vi "animate side opening.vi"(10 "expand/collapse":bool, 11 "Splitter in":refnum<vi>) -> ()   [LabVIEW 2016, in "FPGA RM System Definition API.lvlib"]
uses:
  FPGA-Resource-Manager-APIs/Source/System Definition/FPGA RM System Definition API.lvlib
  visualizer globals.vi
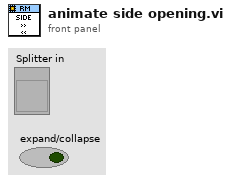
[diagram p1: front panel]
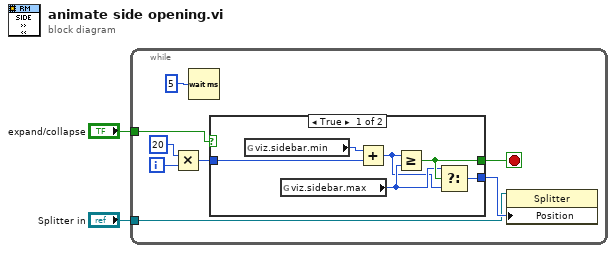
[diagram p0: block diagram]
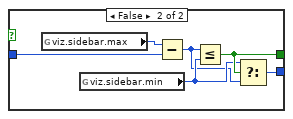
[diagram p2: hidden frame]
diagram:
  n1 = while {
    tunnel: "expand/collapse" -> [w10]
    tunnel: "Splitter in" -> [w3]
    i -> [w6]
    stop <- w9 stop-if-true
    n2 = Multiply(x=20, y=w6) -> (x*y=w5:i32)
    n3 = Wait (ms)(milliseconds to wait=u32 5) -> ()  [unwired: 1 out]
    n4 = case shown="True" w10 {
      tunnel: [w14 w20] -> w9
      tunnel: [w11 w17] -> w8
      tunnel: w5 -> [w16 w22]
      frame True {
        n5 = global read "visualizer globals.vi" "viz.sidebar.min"() -> (w15:i32)
        n6 = global read "visualizer globals.vi" "viz.sidebar.max"() -> (w13:i32)
        n7 = Add(x=w15, y=w16) -> (x+y=w12:i32)
        n8 = Greater Or Equal?(x=w12, y=w13) -> (x >= y?=w14:bool)
        n9 = Select(t=w13, s=w14, f=w12) -> (s? t:f=w11:i32)
      }
      frame False {
        n10 = global read "visualizer globals.vi" "viz.sidebar.max"() -> (w21:i32)
        n11 = global read "visualizer globals.vi" "viz.sidebar.min"() -> (w19:i32)
        n12 = Subtract(x=w21, y=w22) -> (x-y=w18:i32)
        n13 = Less Or Equal?(x=w18, y=w19) -> (x <= y?=w20:bool)
        n14 = Select(t=w19, s=w20, f=w18) -> (s? t:f=w17:i32)
      }
    }
    n15 = property on="Property Node" class="Splitter"(reference=w3, "Position"=w8) -> ()  [unwired: 1 in, 2 out]
  }
